vi "Vision Processing.vi"(4 "error in (no error)":errorcluster, 7 "Image Size":T1=enum."320x240") -> ()   [LabVIEW 2018]
doc: "This VI runs in parallel to other tasks. It gets images from the camera, processes them for color or shape and uses commands or globals to affect the behavior of other subsystems."
uses:
  <vilib>/Rock Robotics/WPI/Camera/WPI_CameraImageSize.ctl
  <vilib>/Rock Robotics/WPI/Camera/WPI_CameraWhite Balance Values.ctl
  <vilib>/Rock Robotics/WPI/Camera/WPI_CameraExposure Values.ctl
  <vilib>/Rock Robotics/WPI/Camera/WPI_CameraFrameRate.ctl
  Framework/Robot Global Data.vi
panel:
  in  "Image Size 2":T1=enum."320x240"
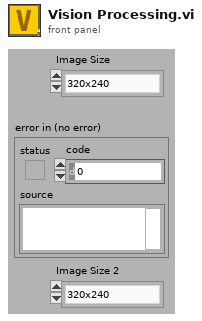
[diagram p1: front panel]
types:
  T1 = typedef "WPI_CameraImageSize.ctl" = enum16{"640x480", "320x240", "160x120", "Custom"}
  T2 = typedef "WPI_CameraFrameRate.ctl" = u32
  T3 = typedef "WPI_CameraExposure Values.ctl" = enum16{"Auto", "Flicker-free 50 Hz", "Flicker-free 60 Hz", "Hold current", "Custom"}
  T4 = typedef "WPI_CameraWhite Balance Values.ctl" = enum16{"Auto", "Fixed indoor", "Fixed outdoor 1", "Fixed outdoor 2", "Fixed fluorescent 1", "Fixed fluorescent 2", "Hold current", "Custom"}
  T5 = typedef "WPI_CameraDevRef.ctl" = cluster{"Camera Address":string, "CameraStatus":errorcluster}
  T6 = typedef "Image Type" = u32
  T7 = typedef "IMAQ Image.ctl" = refnum<image>
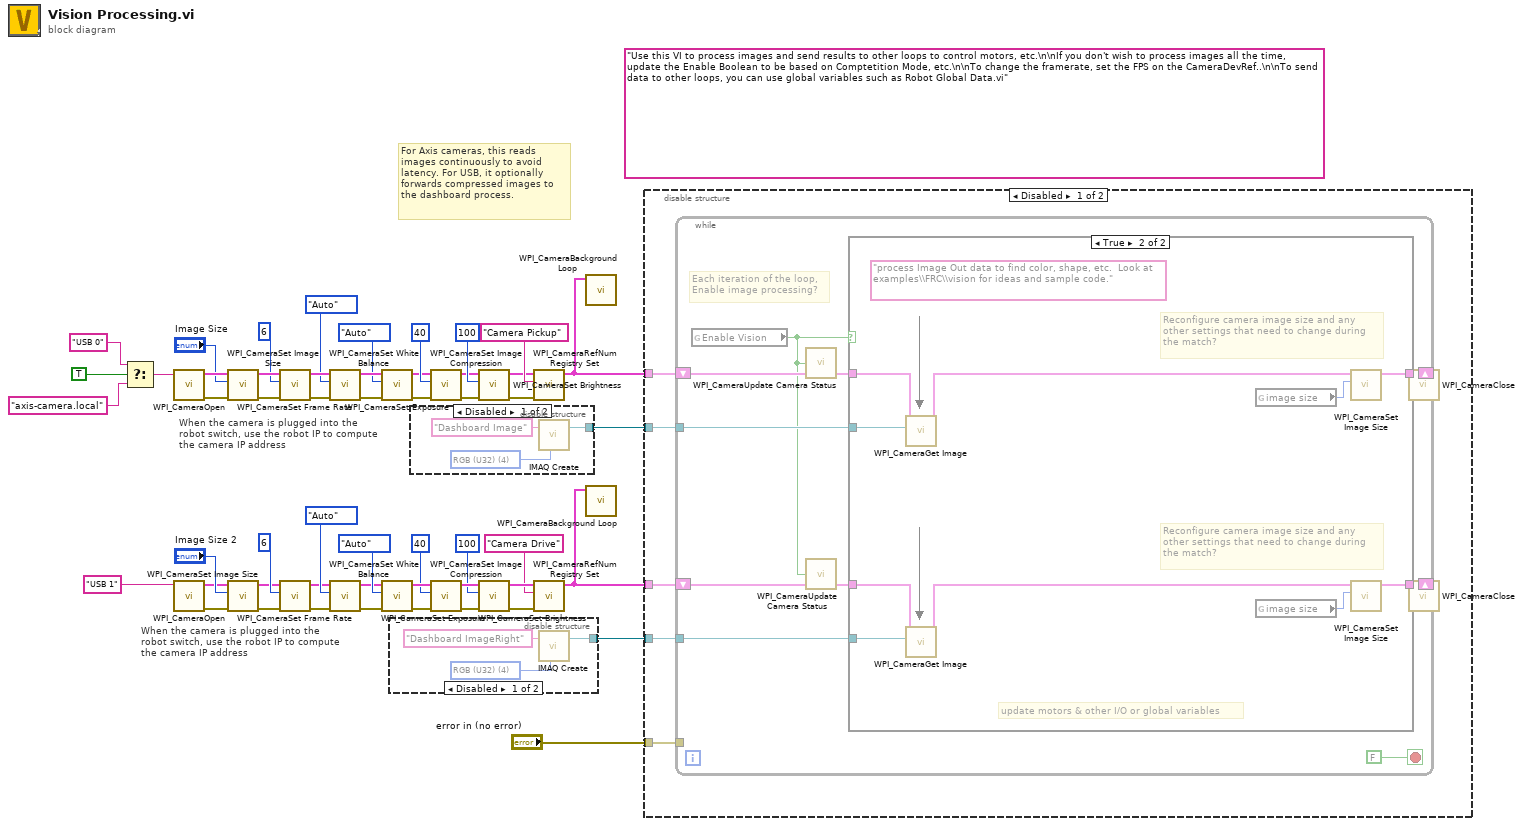
[diagram p0: block diagram]
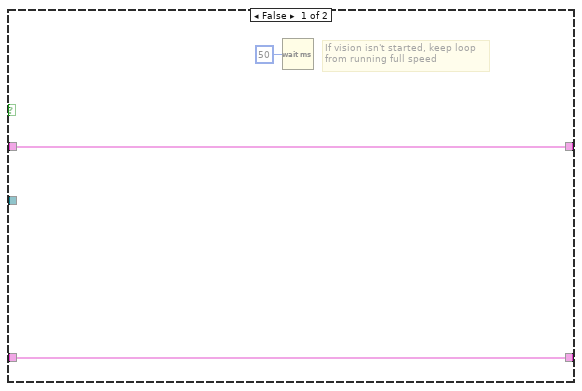
[diagram p4: hidden frame]
diagram:
  (unwired) "Use this VI to process images and send results to other loops to control motors, etc.\n\nIf you don't wish to process images all the time, update the Enable Boolean to be based on Comptetition Mode, etc.\n\nTo change the framerate, set the FPS on the CameraDevRef..\n\nTo send data to other loops, you can use global variables such as Robot Global Data.vi"
  # "When the camera is plugged into the\nrobot switch, use the robot IP to compute\nthe camera IP address"
  # "When the camera is plugged into the\nrobot switch, use the robot IP to compute\nthe camera IP address"
  # "For Axis cameras, this reads\nimages continuously to avoid\nlatency. For USB, it optionally\nforwards compressed images to\nthe dashboard process."
  n1 = Select(t="USB 0" ("format string"), s=TRUE ("dot notation? (F)"), f="axis-camera.local" ("format string")) -> (s? t:f=w26:string)
  n2 = call <vilib>:"WPI_CameraOpen.vi"("Camera Address"=w26) -> ("error out"=w42:errorcluster, "CameraDevRef"=w43:T5)  [unwired: 1 in, 8 out]
  n3 = call <vilib>:"WPI_CameraOpen.vi"("Camera Address"="USB 1" ("format string")) -> ("error out"=w13:errorcluster, "CameraDevRef"=w12:T5)  [unwired: 1 in, 8 out]
  n4 = call <vilib>:"WPI_CameraSet Image Size.vi"("error in (no error)"=w42, "Image Size"="Image Size", "CameraDevRef"=w43) -> ("error out"=w41:errorcluster, "CameraDevRef Out"=w44:T5)  [unwired: 1 in, 6 out]
  n5 = call <vilib>:"WPI_CameraSet Image Size.vi"("error in (no error)"=w13, "Image Size"="Image Size 2", "CameraDevRef"=w12) -> ("error out"=w14:errorcluster, "CameraDevRef Out"=w11:T5)  [unwired: 1 in, 6 out]
  n6 = call <vilib>:"WPI_CameraSet Frame Rate.vi"("error in (no error)"=w41, "Frame Rate (fps)"=T2 6, "CameraDevRef"=w44) -> ("error out"=w40:errorcluster, "CameraDevRef Out"=w46:T5)  [unwired: 7 out]
  n7 = call <vilib>:"WPI_CameraSet Frame Rate.vi"("error in (no error)"=w14, "Frame Rate (fps)"=T2 6, "CameraDevRef"=w11) -> ("error out"=w15:errorcluster, "CameraDevRef Out"=w9:T5)  [unwired: 7 out]
  n8 = call <vilib>:"WPI_CameraSet White Balance.vi"("error in (no error)"=w40, "White Balance"=WPI_CameraWhite_Balance_Values."Auto", "CameraDevRef"=w46) -> ("error out"=w39:errorcluster, "CameraDevRef Out"=w45:T5)  [unwired: 1 in, 6 out]
  n9 = call <vilib>:"WPI_CameraSet White Balance.vi"("error in (no error)"=w15, "White Balance"=WPI_CameraWhite_Balance_Values."Auto", "CameraDevRef"=w9) -> ("error out"=w16:errorcluster, "CameraDevRef Out"=w10:T5)  [unwired: 1 in, 6 out]
  n10 = call <vilib>:"WPI_CameraSet Exposure.vi"("error in (no error)"=w39, "Exposure"=WPI_CameraExposure_Values."Auto", "CameraDevRef"=w45) -> ("error out"=w38:errorcluster, "CameraDevRef Out"=w48:T5)  [unwired: 1 in, 6 out]
  n11 = call <vilib>:"WPI_CameraSet Exposure.vi"("error in (no error)"=w16, "Exposure"=WPI_CameraExposure_Values."Auto", "CameraDevRef"=w10) -> ("error out"=w17:errorcluster, "CameraDevRef Out"=w7:T5)  [unwired: 1 in, 6 out]
  n12 = disable-structure shown="Disabled" {
    disable-tunnel: [w53 _] -> w2
    frame Disabled {
      w54 = T6 4 items=["Grayscale (U8)", "Grayscale (I16)", "Grayscale (SGL)", "Complex (CSG)", "RGB (U32)", "HSL (U32)", "RGB (U64)"] ("Image Type")
      n13 = call "IMAQ Create"("Image Name"="Dashboard ImageRight", "Image Type"=w54) -> ("New Image"=w53:T7)  [unwired: 2 in, 2 out]
    }
    frame Enabled {
    }
  }
  n14 = disable-structure shown="Disabled" {
    disable-tunnel: [w56 _] -> w52
    frame Disabled {
      w58 = T6 4 items=["Grayscale (U8)", "Grayscale (I16)", "Grayscale (SGL)", "Complex (CSG)", "RGB (U32)", "HSL (U32)", "RGB (U64)"] ("Image Type")
      n15 = call "IMAQ Create"("Image Name"="Dashboard Image", "Image Type"=w58) -> ("New Image"=w56:T7)  [unwired: 2 in, 2 out]
    }
    frame Enabled {
    }
  }
  n16 = call <vilib>:"WPI_CameraSet Image Compression.vi"("error in (no error)"=w38, "Compression"=40, "CameraDevRef"=w48) -> ("error out"=w37:errorcluster, "CameraDevRef Out"=w47:T5)  [unwired: 7 out]
  n17 = call <vilib>:"WPI_CameraSet Image Compression.vi"("error in (no error)"=w17, "Compression"=40, "CameraDevRef"=w7) -> ("error out"=w18:errorcluster, "CameraDevRef Out"=w8:T5)  [unwired: 7 out]
  n18 = call <vilib>:"WPI_CameraSet Brightness.vi"("error in (no error)"=w37, "Brightness"=100, "CameraDevRef"=w47) -> ("error out"=w35:errorcluster, "CameraDevRef Out"=w36:T5)  [unwired: 1 in, 6 out]
  n19 = call <vilib>:"WPI_CameraSet Brightness.vi"("error in (no error)"=w18, "Brightness"=100, "CameraDevRef"=w8) -> ("error out"=w20:errorcluster, "CameraDevRef Out"=w19:T5)  [unwired: 1 in, 6 out]
  n20 = call <vilib>:"WPI_CameraRefNum Registry Set.vi"("error in (no error)"=w35, "refnum name"="Camera Pickup", "CameraDevRef"=w36) -> ("CameraDevRef"=w31:T5)  [unwired: 1 in, 7 out]
  n21 = call <vilib>:"WPI_CameraRefNum Registry Set.vi"("error in (no error)"=w20, "refnum name"="Camera Drive", "CameraDevRef"=w19) -> ("CameraDevRef"=w3:T5)  [unwired: 1 in, 7 out]
  n22 = call <vilib>:"WPI_CameraBackground Loop.vi"("CameraDevRef"=w31) -> ()  [unwired: 11 in]
  n23 = call <vilib>:"WPI_CameraBackground Loop.vi"("CameraDevRef"=w3) -> ()  [unwired: 11 in]
  n24 = disable-structure shown="Disabled" {
    disable-tunnel: w52 -> [w65 _]
    disable-tunnel: w31 -> [w64 _]
    disable-tunnel: "error in (no error)" -> [w62 _]
    disable-tunnel: w3 -> [w60 _]
    disable-tunnel: w2 -> [w59 _]
    frame Disabled {
      n25 = while {
        shift-right: [w74] -> w63
        shift-left: w64 -> [w72]
        tunnel: w65 -> [w73]
        tunnel: w62 -> [_]
        shift-right: [w68] -> w61
        shift-left: w60 -> [w69]
        tunnel: w59 -> [w67]
        stop <- FALSE stop-if-true
        # "Each iteration of the loop,\nEnable image processing?"
        n26 = global read "Robot Global Data.vi" "Enable Vision"() -> (w66:bool)
        n27 = call <vilib>:"WPI_CameraUpdate Camera Status.vi"("CameraDevRef In"=w72, "Enable Vision"=w66) -> ("CameraDevRef Out"=w71:T5)  [unwired: 3 in]
        n28 = call <vilib>:"WPI_CameraUpdate Camera Status.vi"("CameraDevRef In"=w69, "Enable Vision"=w66) -> ("CameraDevRef Out"=w70:T5)  [unwired: 3 in]
        n29 = case shown="True" w66 {
          tunnel: w73 -> [_ w87]
          tunnel: [w78 w88] -> w74
          tunnel: w71 -> [w78 w85]
          tunnel: w67 -> [_ w80]
          tunnel: [w76 w79] -> w68
          tunnel: w70 -> [w76 w82]
          frame False {
            # "If vision isn't started, keep loop\nfrom running full speed"
            n30 = Wait (ms)(milliseconds to wait=u32 50) -> ()  [unwired: 1 out]
          }
          frame True {
            (unwired) "process Image Out data to find color, shape, etc.  Look at examples\\FRC\\vision for ideas and sample code."
            # "Reconfigure camera image size and any\nother settings that need to change during\nthe match?"
            # "update motors & other I/O or global variables"
            # "Reconfigure camera image size and any\nother settings that need to change during\nthe match?"
            n31 = call <vilib>:"WPI_CameraGet Image.vi"("Image"=w87, "CameraDevRef"=w85) -> ("CameraDevRef Out"=w84:T5)  [unwired: 1 in, 8 out]
            n32 = call <vilib>:"WPI_CameraGet Image.vi"("Image"=w80, "CameraDevRef"=w82) -> ("CameraDevRef Out"=w83:T5)  [unwired: 1 in, 8 out]
            n33 = global read "Robot Global Data.vi" "image size"() -> (w86:T1)
            n34 = global read "Robot Global Data.vi" "image size"() -> (w81:T1)
            n35 = call <vilib>:"WPI_CameraSet Image Size.vi"("Image Size"=w86, "CameraDevRef"=w84) -> ("CameraDevRef Out"=w88:T5)  [unwired: 2 in, 7 out]
            n36 = call <vilib>:"WPI_CameraSet Image Size.vi"("Image Size"=w81, "CameraDevRef"=w83) -> ("CameraDevRef Out"=w79:T5)  [unwired: 2 in, 7 out]
          }
        }
      }
      n37 = call <vilib>:"WPI_CameraClose.vi"("CameraDevRef"=w63) -> ()  [unwired: 1 in, 10 out]
      n38 = call <vilib>:"WPI_CameraClose.vi"("CameraDevRef"=w61) -> ()  [unwired: 1 in, 10 out]
    }
    frame Enabled {
    }
  }
